vi "setConfigArray.vi"(8 "error in (no error)":errorcluster, 10 "ConfigArray":T1(array[cluster]), 11 "EthernetSupply in":refnum<class "ethernetSupply.lvclass">) -> (0 "error out":errorcluster, 3 "EthernetSupply out":refnum<class "ethernetSupply.lvclass">)   [LabVIEW 2011, in "Tools.lvlib" / "DatabaseHelpers.lvlib" / "ethernetSupply.lvclass"]
uses:
  ethernetSupply.lvclass
  ethernetSupply.lvclass/ethernetSupply.ctl
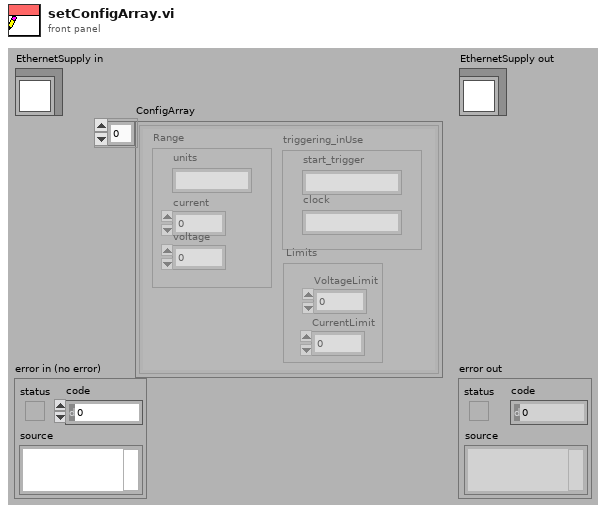
[diagram p1: front panel]
types:
  T1 = cluster{"Range":cluster{"units":string, "current":dbl, "voltage":dbl}, "triggering_inUse":cluster{"start_trigger":string, "clock":string}, "Limits":cluster{"VoltageLimit":dbl, "CurrentLimit":dbl}}[]
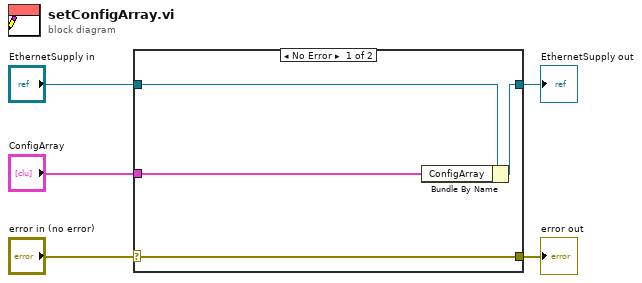
[diagram p0: block diagram]
diagram:
  n1 = case shown="No Error" "error in (no error)" {
    selector: "error in (no error)" -> [w9 w10]
    tunnel: [w9 w10] -> w4
    tunnel: [w7 w11] -> w2
    tunnel: "EthernetSupply in" -> [w8 w11]
    tunnel: "ConfigArray" -> [w6 _]
    frame No Error {
      n2 = Bundle By Name(cluster=w8, "ConfigArray"=w6) -> (w7:refnum<class "ethernetSupply.lvclass">)
    }
    frame Error {
    }
  }
  "error out" <- w4
  "EthernetSupply out" <- w2
